vi "SendReq.vi"(1 "Param":u32, 4 "MsgId":u8) -> ()   [LabVIEW 2016]
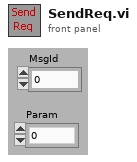
[diagram p1: front panel]
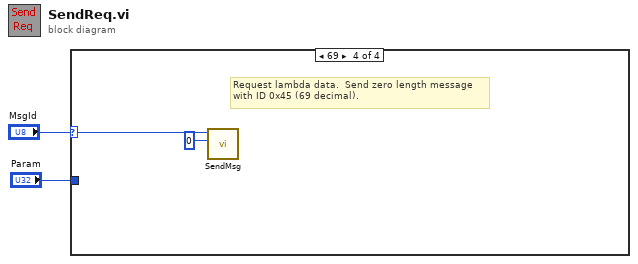
[diagram p0: block diagram]
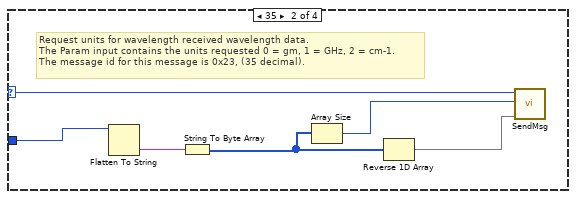
[diagram p3: hidden frame]
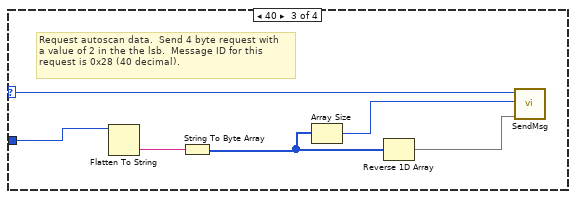
[diagram p4: hidden frame]
diagram:
  n1 = case shown="69" "MsgId" {
    selector: "MsgId" -> [_ w8 w14 w15]
    tunnel: "Param" -> [_ w3 w9 _]
    frame 0, Default {
    }
    frame 35 {
      # "Request units for wavelength received wavelength data.\nThe Param input contains the units requested 0 = gm, 1 = GHz, 2 = cm-1.\nThe message id for this message is 0x23, (35 decimal)."
      n2 = Flatten To String(anything=w3) -> (data string=w7:string)  [unwired: 3 in, 2 out]
      n3 = String To Byte Array(string=w7) -> (unsigned byte array=w5:u8[])
      n4 = Array Size(array=w5) -> (size(s)=w6:i32)
      n5 = Reverse 1D Array(array=w5) -> (reversed array=w4:u8[])
      n6 = call "SendMsg.vi"("Body"=w4, "Length"=w6, "ID"=w8) -> ()  [unwired: 2 in]
    }
    frame 40 {
      # "Request autoscan data.  Send 4 byte request with\na value of 2 in the the lsb.  Message ID for this\nrequest is 0x28 (40 decimal)."
      n7 = Flatten To String(anything=w9) -> (data string=w13:string)  [unwired: 3 in, 2 out]
      n8 = String To Byte Array(string=w13) -> (unsigned byte array=w11:u8[])
      n9 = Array Size(array=w11) -> (size(s)=w12:i32)
      n10 = Reverse 1D Array(array=w11) -> (reversed array=w10:u8[])
      n11 = call "SendMsg.vi"("Body"=w10, "Length"=w12, "ID"=w14) -> ()  [unwired: 2 in]
    }
    frame 69 {
      # "Request lambda data.  Send zero length message\nwith ID 0x45 (69 decimal)."
      n12 = call "SendMsg.vi"("Length"=u16 0, "ID"=w15) -> ()  [unwired: 3 in]
    }
  }
